vi "PH_AxisGUI_6P.PC_Reset.vi"(0 "i ref in":refnum<vi>, 2 "AxisSelection":enum32{"Axis1", "Axis2", "Both"}(ring), 5 "error in":errorcluster) -> (14 "i ref out":refnum<vi>, 19 "error out":errorcluster)   [LabVIEW 2014]
uses:
  PH_AxisGUI_6P.lvlib
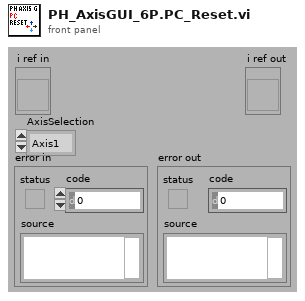
[diagram p1: front panel]
types:
  T1 = typedef "PH_AxisGUI_BaseClass.lvlib/PH_AxisGUI_BaseClass.Dataset In Constructor.ctl" = cluster{"Address":T2, "Name":string, "Label \"Back\"":string, "Labell \"Forth\"":string}
  T2 = typedef "PH_Motion.Axis Address.ctl" = cluster{"Instance":string, "Motor Nr":i32}
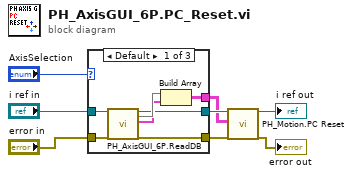
[diagram p0: block diagram]
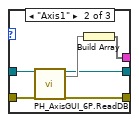
[diagram p2: hidden frame]
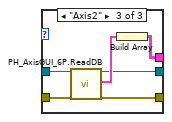
[diagram p3: hidden frame]
diagram:
  n1 = case shown="Default" "AxisSelection" {
    tunnel: [w9 w16 w23] -> w3
    tunnel: [w10 w17 w22] -> w6
    tunnel: "error in" -> [w15 w21 w26]
    tunnel: "i ref in" -> [w14 w20 w27]
    tunnel: [w11 w18 w25] -> w1
    frame Default {
      n2 = call "PH_AxisGUI_6P.ReadDB.vi"("i ref in"=w14, "error in (no error)"=w15) -> ("i ref out"=w9:refnum<vi>, 15:w13, "Data In Base Axis GUI Constructor"=w12:T1[], "error out"=w10:errorcluster)  [unwired: 14 in]
      n3 = Build Array(w13, w12) -> (w11:T1[][])
    }
    frame "Axis1" {
      n4 = call "PH_AxisGUI_6P.ReadDB.vi"("i ref in"=w20, "error in (no error)"=w21) -> ("i ref out"=w16:refnum<vi>, 15:w19, "error out"=w17:errorcluster)  [unwired: 14 in, 1 out]
      n5 = Build Array(w19) -> (w18:void[])
    }
    frame "Axis2" {
      n6 = call "PH_AxisGUI_6P.ReadDB.vi"("i ref in"=w27, "error in (no error)"=w26) -> ("i ref out"=w23:refnum<vi>, "Data In Base Axis GUI Constructor"=w24:T1[], "error out"=w22:errorcluster)  [unwired: 15 in]
      n7 = Build Array(w24) -> (w25:T1[][])
    }
  }
  n8 = call "PH_Motion.PC Reset.vi"("VI in"=w3, "Addresses"=w1, "error in (no error)"=w6) -> ("VI out"=→"i ref out":refnum<vi>, "error out"=→"error out":errorcluster)  [unwired: 15 in]
